vi "Get Travel Units.vi"(8 "error in (no error)":errorcluster, 11 "ESM303 in":refnum<class "ESM303.lvclass">) -> (0 "error out":errorcluster, 2 "Travel Units":T1, 3 "ESM303 out":refnum<class "ESM303.lvclass">)   [LabVIEW 2018, in "ESM303.lvlib" / "ESM303.lvclass"]
uses:
  ESM303.lvclass
  builds/Force Test Stand/Force Test Stand/Force Test Stand.lvlibp/Custom Controls/Speed Units.ctl
  builds/Force Test Stand/Force Test Stand/Force Test Stand.lvlibp/Force Test Stand.lvclass
  C:/Projects/LabVIEW/In-Progress/Jose Rivero-Diaz/builds/Force Test Stand/Force Test Stand/Force Test Stand.lvlibp/Force Test Stand.lvclass
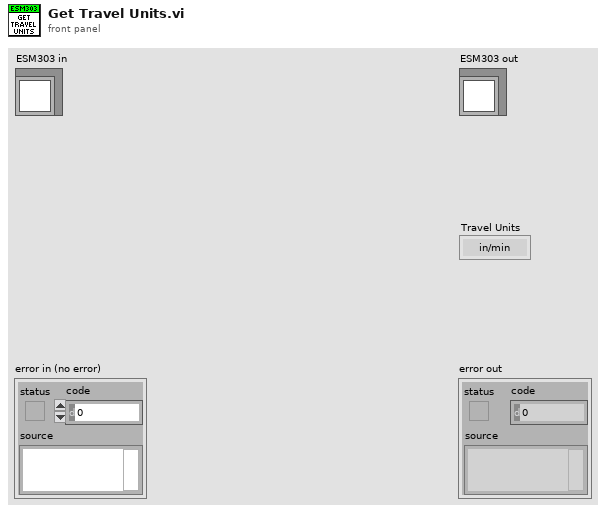
[diagram p1: front panel]
types:
  T1 = typedef "Force Test Stand.lvlibp/Force Test Stand.lvclass/Speed Units.ctl" = enum16{"in/min", "mm/min"}
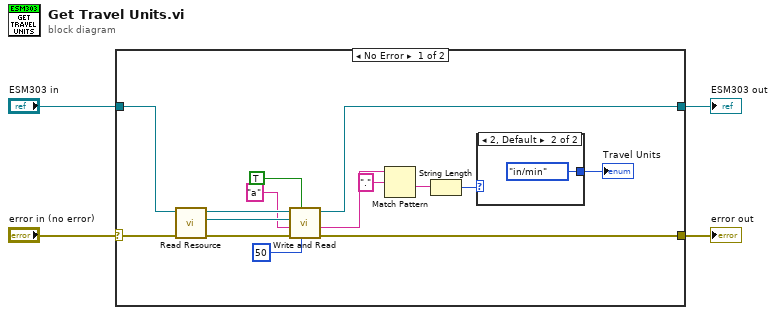
[diagram p0: block diagram]
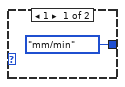
[diagram p2: hidden frame]
diagram:
  n1 = case shown="No Error" "error in (no error)" {
    selector: "error in (no error)" -> [w19 w22]
    tunnel: [w11 w23] -> w3
    tunnel: "ESM303 in" -> [w18 w23]
    tunnel: [w10 w22] -> w1
    frame No Error {
      n2 = call "Read Resource.vi"("error in (no error)"=w19, "Force Test Stand in"=w18) -> ("error out"=w15:errorcluster, "Resource"=w16:refnum<visa-resource-name>, "Force Test Stand out"=w17:refnum<class "ESM303.lvclass">)  [unwired: 7 in]
      n3 = call "Write and Read.vi"("Delay Before Read (ms)"=50, "Write & Read"=TRUE, "error in (no error)"=w15, "Command"="a", "VISA Refnum in"=w16, "ESM303 in"=w17) -> ("error out"=w10:errorcluster, "Response"=w8:string, "ESM303 out"=w11:refnum<class "ESM303.lvclass">)  [unwired: 3 in]
      n4 = Match Pattern(string=w8, regular expression=".") -> (after substring=w6:string)  [unwired: 1 in, 3 out]
      n5 = String Length(string=w6) -> (length=w5:i32)
      n6 = case shown="2, Default" w5 {
        tunnel: [Speed_Units."mm/min" ("Speed Units") Speed_Units."in/min" ("Speed Units")] -> w9
        frame 1 {
        }
        frame 2, Default {
        }
      }
      "Travel Units" <- w9
    }
    frame Error {
    }
  }
  "error out" <- w1
  "ESM303 out" <- w3
